vi "WristStartPosition.vi"(8 "error in (no error)":errorcluster) -> (0 "error out":errorcluster, 3 "Numeric":dbl)   [LabVIEW 2023]
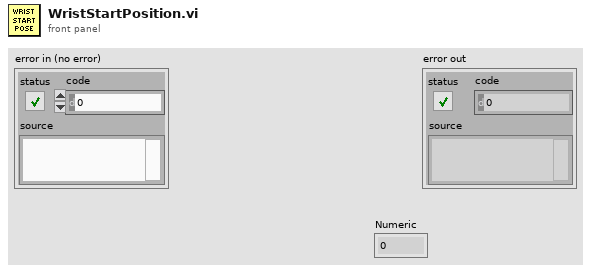
[diagram p1: front panel]
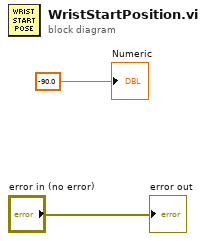
[diagram p0: block diagram]
diagram:
  "Numeric" <- -90.0 ("Numeric")
  "error out" <- "error in (no error)"
